vi "simple pulse train filter.vi"(9 "filter params":T1={"filterSize"=50, "lowerThreshold"=5, "upperThreshold"=45}, 11 "realState":bool=TRUE) -> (3 "filteredState":bool)   [LabVIEW 2018]
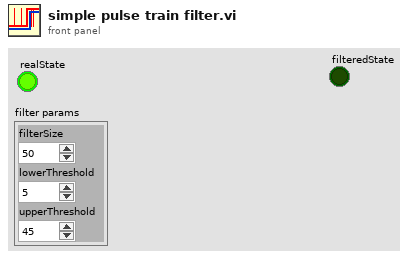
[diagram p1: front panel]
types:
  T1 = cluster{"filterSize":i16, "lowerThreshold":u8, "upperThreshold":u8}
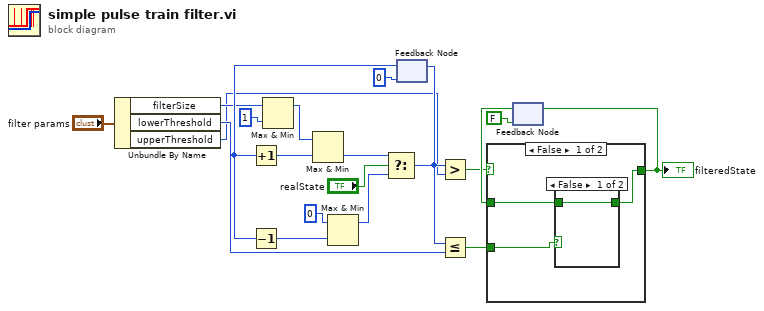
[diagram p0: block diagram]
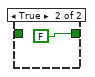
[diagram p2: hidden frame]
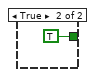
[diagram p3: hidden frame]
diagram:
  n1 = Unbundle By Name("filter params") -> ("filterSize"=w3:i16, "lowerThreshold"=w2:u8, "upperThreshold"=w1:u8)
  n2 = Max & Min(x=w3, y=u8 1) -> (max(x,y)=w6:i16)  [unwired: 1 out]
  n3 = feedback #1(u8 0) -> (w14:i16)
  n4 = Increment(x=w14) -> (x+1=w19:i16)
  n5 = Decrement(x=w14) -> (x-1=w17:i16)
  n6 = Max & Min(x=w6, y=w19) -> (min(x,y)=w18:i16)  [unwired: 1 out]
  n7 = Max & Min(x=u8 0 ("filterSize"), y=w17) -> (max(x,y)=w16:i16)  [unwired: 1 out]
  n8 = Select(t=w18, s="realState", f=w16) -> (s? t:f=w8:i16)
  n9 = feedback-in #1(w8) -> ()
  n10 = Greater?(x=w8, y=w1) -> (0:w11:bool)
  n11 = Less Or Equal?(x=w8, y=w2) -> (x <= y?=w10:bool)
  n12 = feedback #2(FALSE ("state")) -> (w12:bool)
  n13 = case shown="False" w11 {
    tunnel: w12 -> [w21 _]
    tunnel: [w22 TRUE] -> w9
    tunnel: w10 -> [w23 _]
    frame False {
      n14 = case shown="False" w23 {
        tunnel: [w24 FALSE] -> w22
        tunnel: w21 -> [w24 _]
        frame False {
        }
        frame True {
        }
      }
    }
    frame True {
    }
  }
  "filteredState" <- w9
  n15 = feedback-in #2(w9) -> ()
